vi "SGLMultiply.vi"() -> ()   [LabVIEW 2016]
uses:
  Accelerometer/AccelerometerSample.ctl
  <vilib>/rvi/Emulation/niFpgaGetClockAttributes.vi
  <vilib>/rvi/Emulation/niFpgaSctlEmulationGetInTimedLoop.vi
  <vilib>/rvi/Emulation/niFpgaEmulationReportErrorSimple.vi
  <vilib>/rvi/Emulation/niFpgaEmulationIsFPGAContextNoSignature.vi
  <vilib>/rvi/errors/niFpgaSetErrorForExecOnDevCompSimple.vi
  <vilib>/rvi/eio/common/nirviEmuReportErrorAndStop.vi
  <vilib>/rvi/DataTransferAndStorage/Container/Common/niFpgaContainerGetUniqueNameForEmu.vi
  <vilib>/rvi/FIFO/Fifo_Resource/nirvififoEmulationSetSize.vi
  <vilib>/rvi/FIFO/Fifo_Resource/nirviFifoEmulationQueueMgr.vi
  <instcachedir>/0/nirviFifoEmulationQueueMgr_E5CAEC123FF24DC58D834DCA3CDAA9B5.lvgen/nirviFifoEmulationQueueMgr_E5CAEC123FF24DC58D834DCA3CDAA9B5_026.vi
  <vilib>/Utility/error.llb/Clear Errors.vi
  <vilib>/rvi/FIFO/Fifo_Resource/nirvififoEmulationCreateLock.vi
  <vilib>/rvi/Emulation/niFpgaProcessEmulError.vi
  <vilib>/rvi/FIFO/Fifo_Resource/nirvififoEmulationObtainLock.vi
  <vilib>/rvi/FIFO/Fifo_Resource/nirvififoEmulationReleaseLock.vi
  <vilib>/rvi/occurrence/nirviWaitOnOccurrenceBase.vi
  <vilib>/rvi/errors/nirviReportUnexpectedCaseInternalError.vi
  <vilib>/rvi/errors/nirviReportUnexpectedCaseInternalError (U32).vi
  <userlib>/_NI FLP Library/FPGA/outsideSCTL/FlpLib Multiply Shared Instance 0.vi
  <vilib>/rvi/Emulation/niFpgaCriticalErrorInLSC.vi
  <instcachedir>/0/nirviFifoEmulationQueueMgr_E5CAEC123FF24DC58D834DCA3CDAA9B5.lvgen/nirviFifoEmulationQueueMgr_E5CAEC123FF24DC58D834DCA3CDAA9B5_004.vi
  <vilib>/rvi/FIFO/Fifo_Resource/nirvififoEmulationDetermineInputValidOut.vi
  <vilib>/rvi/DataTransferAndStorage/Container/XNode/niFpgaContainer.xnode
  <vilib>/rvi/FIFO/Fifo_Resource/nirvififoEmulationRead.vi
  <vilib>/rvi/FIFO/Fifo_Resource/nirvififoEmulationWrite.vi
panel:
  out "output cluster":T1
  in  "Voltage5":sgl=3.200729
  in  "Voltage6":sgl=-3.200611
  in  "Voltage7":sgl=4.200899
  in  "Voltage8":sgl=-1.200478
  in  "Voltage4":sgl=-2.200018
  in  "Voltage3":sgl=2.202255
  in  "Voltage2":sgl=-1.199524
  in  "Voltage1":sgl=1.200108
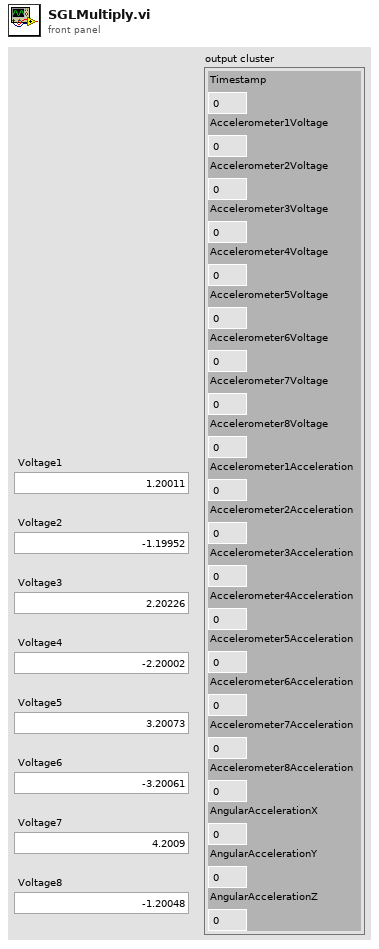
[diagram p1: front panel]
types:
  T1 = typedef "AccelerometerSample.ctl" = cluster{"Timestamp":u64, "Accelerometer1Voltage":sgl, "Accelerometer2Voltage":sgl, "Accelerometer3Voltage":sgl, "Accelerometer4Voltage":sgl, "Accelerometer5Voltage":sgl, "Accelerometer6Voltage":sgl, "Accelerometer7Voltage":sgl, "Accelerometer8Voltage":sgl, "Accelerometer1Acceleration":sgl, "Accelerometer2Acceleration":sgl, "Accelerometer3Acceleration":sgl, "Accelerometer4Acceleration":sgl, "Accelerometer5Acceleration":sgl, "Accelerometer6Acceleration":sgl, "Accelerometer7Acceleration":sgl, "Accelerometer8Acceleration":sgl, "AngularAccelerationX":sgl, "AngularAccelerationY":sgl, "AngularAccelerationZ":sgl}
  T2 = cluster{"Timestamp":u64, "Accelerometer1Voltage":sgl, "Accelerometer2Voltage":sgl, "Accelerometer3Voltage":sgl, "Accelerometer4Voltage":sgl, "Accelerometer5Voltage":sgl, "Accelerometer6Voltage":sgl, "Accelerometer7Voltage":sgl, "Accelerometer8Voltage":sgl, "Accelerometer1Acceleration":sgl, "Accelerometer2Acceleration":sgl, "Accelerometer3Acceleration":sgl, "Accelerometer4Acceleration":sgl, "Accelerometer5Acceleration":sgl, "Accelerometer6Acceleration":sgl, "Accelerometer7Acceleration":sgl, "Accelerometer8Acceleration":sgl, "AngularAccelerationX":sgl, "AngularAccelerationY":sgl, "AngularAccelerationZ":sgl}
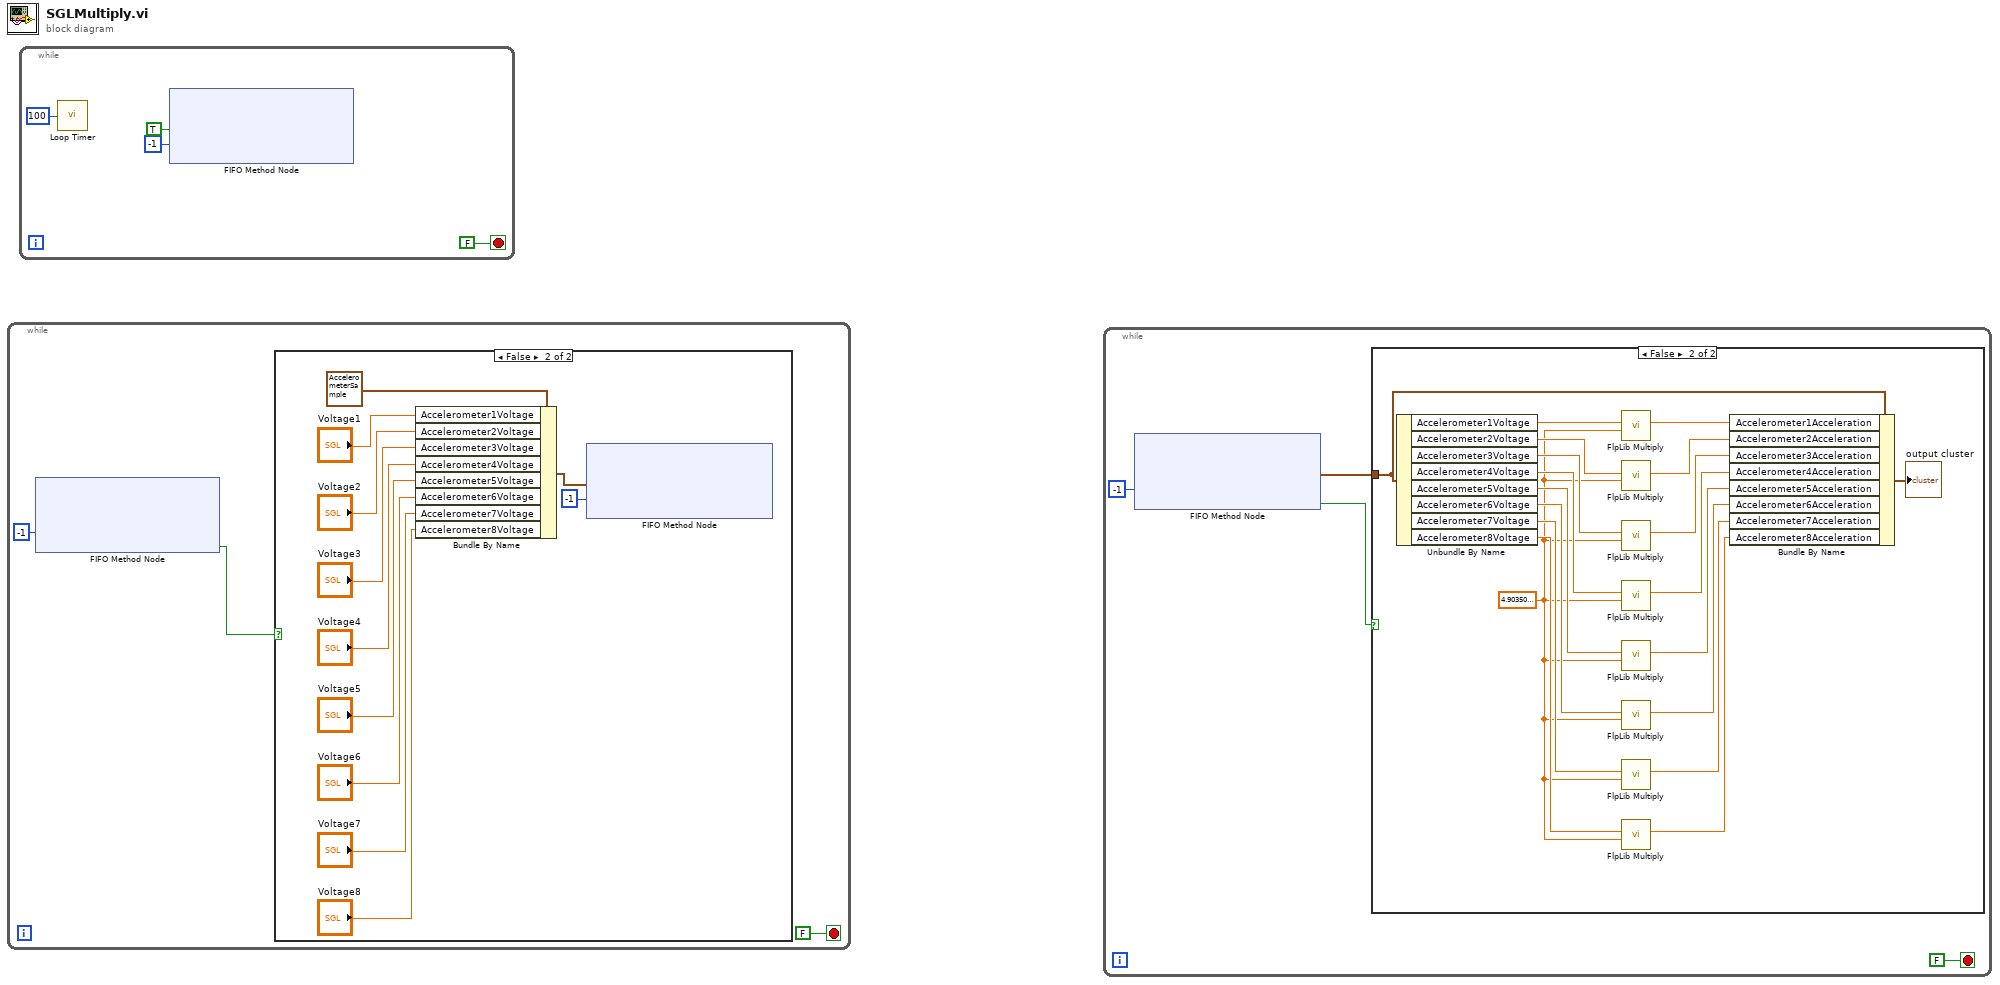
[diagram p0: block diagram]
diagram:
  n1 = while {
    stop <- FALSE stop-if-true
    n2 = xnode ("FIFO Method Node")("Timeout"=-1) -> ("Timed Out?"=w2:bool)  [unwired: 1 in, 2 out]
    n3 = case shown="False" w2 {
      frame True {
      }
      frame False {
        n4 = Bundle By Name(cluster=T1 {"Timestamp"=0, "Accelerometer1Voltage"=0.0, "Accelerometer2Voltage"=0.0, "Accelerometer3Voltage"=0.0, "Accelerometer4Voltage"=0.0, "Accelerometer5Voltage"=0.0, "Accelerometer6Voltage"=0.0, "Accelerometer7Voltage"=0.0, "Accelerometer8Voltage"=0.0, "Accelerometer1Acceleration"=0.0, "Accelerometer2Acceleration"=0.0, "Accelerometer3Acceleration"=0.0, "Accelerometer4Acceleration"=0.0, "Accelerometer5Acceleration"=0.0, "Accelerometer6Acceleration"=0.0, "Accelerometer7Acceleration"=0.0, "Accelerometer8Acceleration"=0.0, "AngularAccelerationX"=0.0, "AngularAccelerationY"=0.0, "AngularAccelerationZ"=0.0} ("AccelerometerSample"), "Accelerometer1Voltage"="Voltage1", "Accelerometer2Voltage"="Voltage2", "Accelerometer3Voltage"="Voltage3", "Accelerometer4Voltage"="Voltage4", "Accelerometer5Voltage"="Voltage5", "Accelerometer6Voltage"="Voltage6", "Accelerometer7Voltage"="Voltage7", "Accelerometer8Voltage"="Voltage8") -> (w5:T1)
        n5 = xnode ("FIFO Method Node")("Element"=w5, "Timeout"=-1) -> ()  [unwired: 1 in, 2 out]
      }
    }
  }
  n6 = while {
    stop <- FALSE stop-if-true
    n7 = call "Loop Timer"("Count(mSec)"=u32 100) -> ()  [unwired: 1 out]
    n8 = xnode ("FIFO Method Node")("Element"=TRUE, "Timeout"=-1) -> ()  [unwired: 1 in, 2 out]
  }
  n9 = while {
    stop <- FALSE stop-if-true
    n10 = xnode ("FIFO Method Node")("Timeout"=-1) -> ("Element"=w21:T2, "Timed Out?"=w19:bool)  [unwired: 1 in, 1 out]
    n11 = case shown="False" w19 {
      tunnel: w21 -> [_ w23]
      frame True {
      }
      frame False {
        w33 = sgl 4.9035 ("y")
        n12 = Unbundle By Name(w23) -> ("Accelerometer1Voltage"=w41:sgl, "Accelerometer2Voltage"=w34:sgl, "Accelerometer3Voltage"=w35:sgl, "Accelerometer4Voltage"=w36:sgl, "Accelerometer5Voltage"=w37:sgl, "Accelerometer6Voltage"=w38:sgl, "Accelerometer7Voltage"=w39:sgl, "Accelerometer8Voltage"=w40:sgl)
        n13 = call-poly <userlib>:"FlpLib Multiply.vi"("y"=w33, "x"=w41) -> ("x*y"=w32:sgl)  [unwired: 5 in]
        n14 = call-poly <userlib>:"FlpLib Multiply.vi"("y"=w33, "x"=w34) -> ("x*y"=w25:sgl)  [unwired: 5 in]
        n15 = call-poly <userlib>:"FlpLib Multiply.vi"("y"=w33, "x"=w35) -> ("x*y"=w26:sgl)  [unwired: 5 in]
        n16 = call-poly <userlib>:"FlpLib Multiply.vi"("y"=w33, "x"=w36) -> ("x*y"=w27:sgl)  [unwired: 5 in]
        n17 = call-poly <userlib>:"FlpLib Multiply.vi"("y"=w33, "x"=w37) -> ("x*y"=w28:sgl)  [unwired: 5 in]
        n18 = call-poly <userlib>:"FlpLib Multiply.vi"("y"=w33, "x"=w38) -> ("x*y"=w29:sgl)  [unwired: 5 in]
        n19 = call-poly <userlib>:"FlpLib Multiply.vi"("y"=w33, "x"=w39) -> ("x*y"=w30:sgl)  [unwired: 5 in]
        n20 = call-poly <userlib>:"FlpLib Multiply.vi"("y"=w33, "x"=w40) -> ("x*y"=w31:sgl)  [unwired: 5 in]
        n21 = Bundle By Name(cluster=w23, "Accelerometer1Acceleration"=w32, "Accelerometer2Acceleration"=w25, "Accelerometer3Acceleration"=w26, "Accelerometer4Acceleration"=w27, "Accelerometer5Acceleration"=w28, "Accelerometer6Acceleration"=w29, "Accelerometer7Acceleration"=w30, "Accelerometer8Acceleration"=w31) -> (→"output cluster":T2)
      }
    }
  }
